vi "Run.vi"(8 "error in (no error)":errorcluster, 11 "Channel GUI in":refnum<class "Channel.lvclass">) -> (0 "error out":errorcluster, 3 "Channel GUI out":refnum<class "Channel.lvclass">)   [LabVIEW 2018, in "Channel.lvclass"]
uses:
  Channel.lvclass
  Channel.lvclass/Channel.ctl
  State Machine/State Machine.lvclass
  Camera/Camera.lvclass
  RxTx/RxTx.lvclass
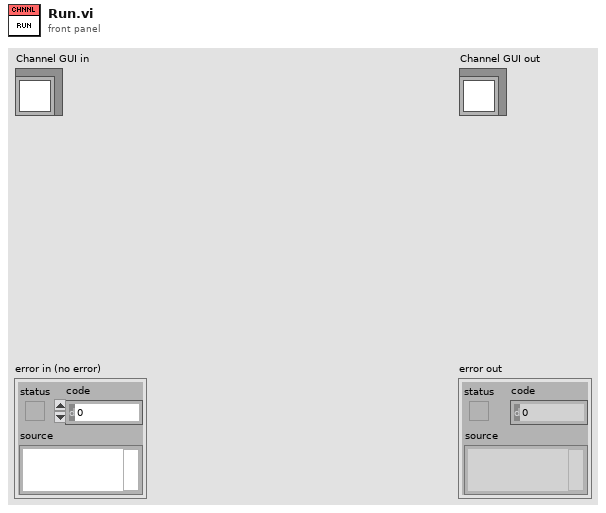
[diagram p1: front panel]
types:
  T1 = cluster{"PREAMP":u16, "READOUT_RATE":u16, "VERTICAL_SHIFT_SPEED":u16, "READ_MODE":u16, "VERTICAL_CLOCK_VOLTAGE":u16, "ACQUISITION_MODE":u16, "AD_CHANNEL":u16, "SHUTTER_TTL":u16, "SHUTTER_OPENING_TIME":u16, "SHUTTER_CLOSING_TIME":u16, "SHUTTER_MODE":u16, "TRIGGER_MODE":u16, "VBIN":u16, "INITIAL_LINE":u16, "INITIAL_COLUMN":u16, "FINAL_LINE":u16, "FINAL_COLUMN":u16, "HBIN":u16}
  T2 = cluster{"EXPTIME":dbl, "#FRAMES":u32, "#CYCLES":u32, "suffix":string, "TEMP":i32, "COOLER_POWER_STATUS":u16}
  T3 = cluster{"CYCLES_DONE":u16, "LAST_IMAGE_NAME":string, "USED_DISK_SPACE":u16, "FRAMES_DONE":u16, "CCD_STATUS":string, "CURRENT_TEMPERATURE":i16, "TEMPERATURE_STATUS":string, "FRAME_EXPOSURE_TIME":sgl, "ERROR":bool, "SERIAL_NUMBER":u16, "ACQUIRING":bool, "IMAGE_INDEX":u32, "power":bool, "acs mode":bool}
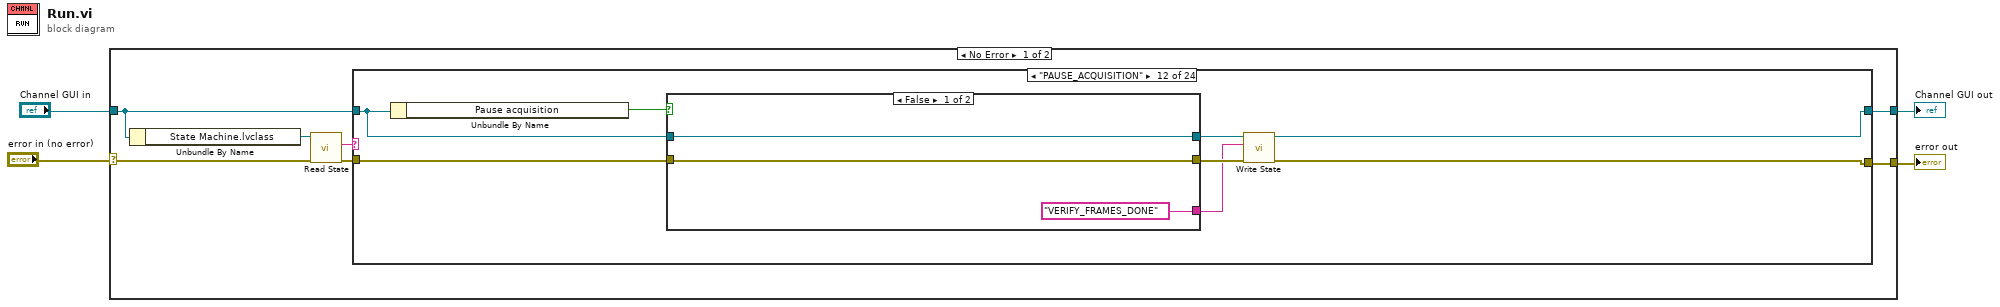
[diagram p0: block diagram]
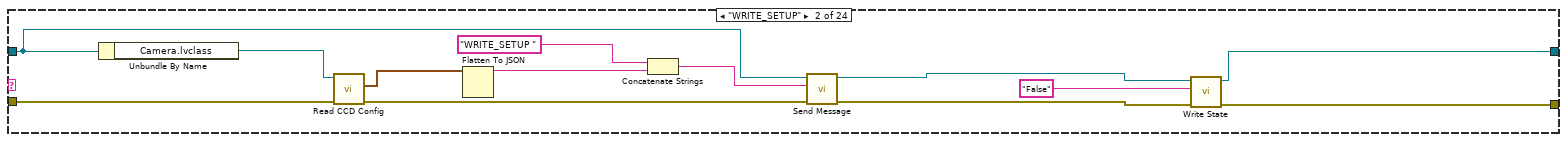
[diagram p3: hidden frame]
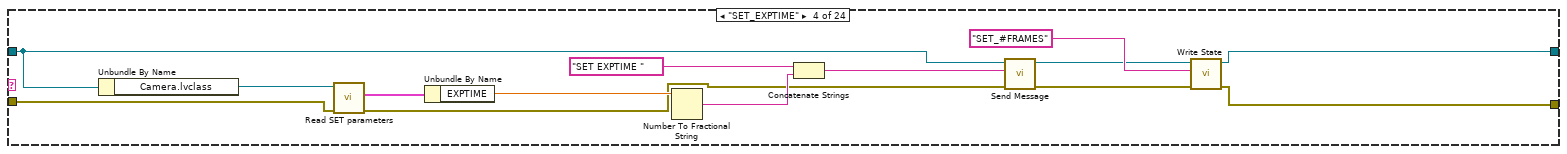
[diagram p5: hidden frame]
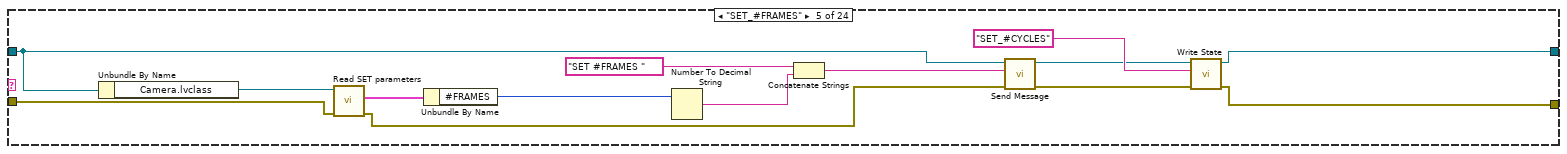
[diagram p6: hidden frame]
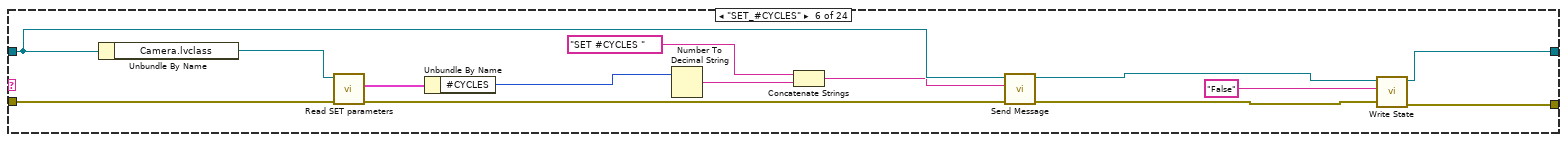
[diagram p7: hidden frame]
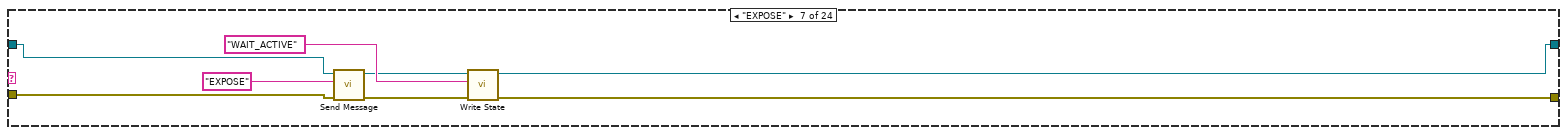
[diagram p8: hidden frame]
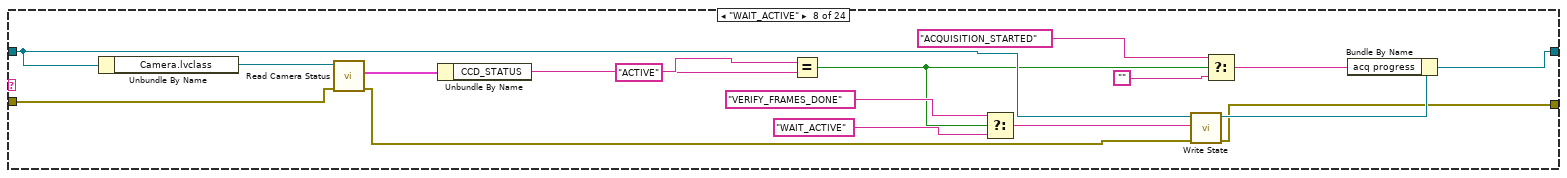
[diagram p9: hidden frame]
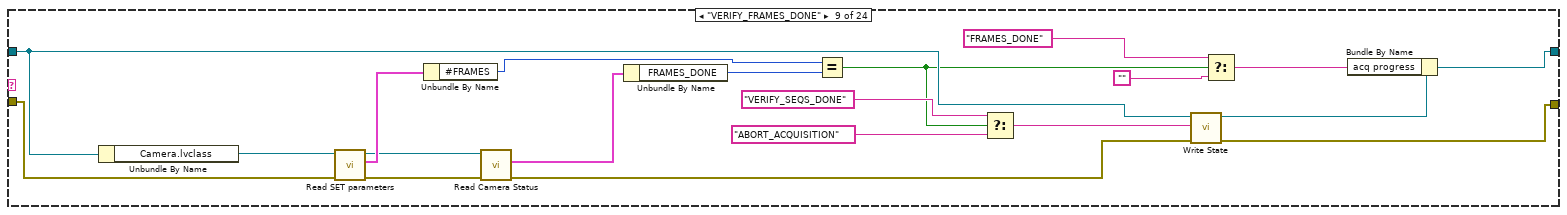
[diagram p10: hidden frame]
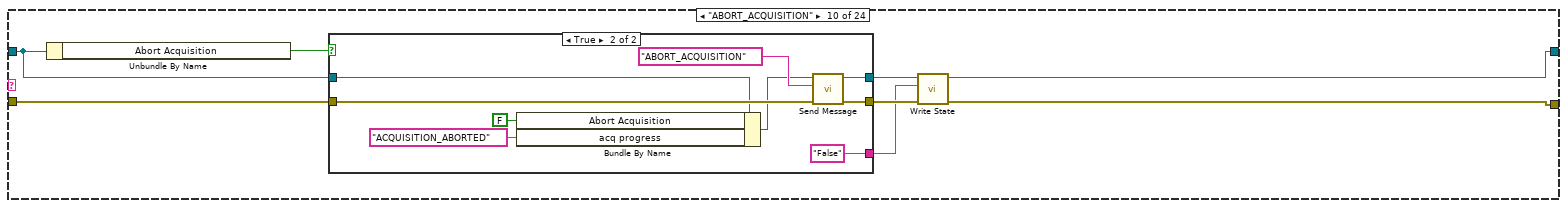
[diagram p11: hidden frame]
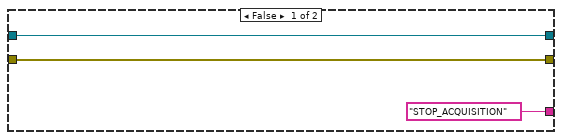
[diagram p12: hidden frame]
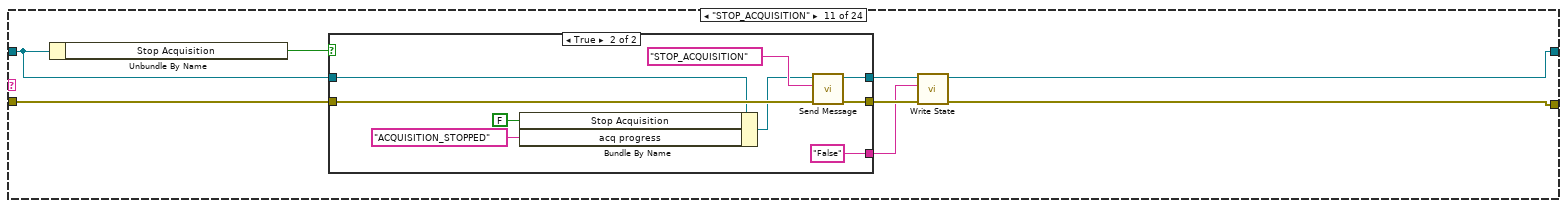
[diagram p13: hidden frame]
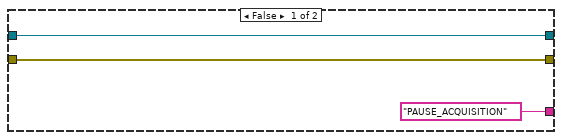
[diagram p14: hidden frame]
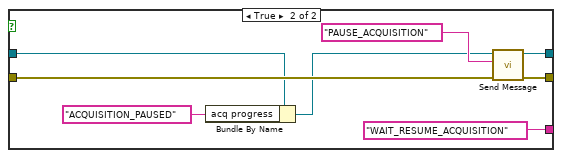
[diagram p15: hidden frame]
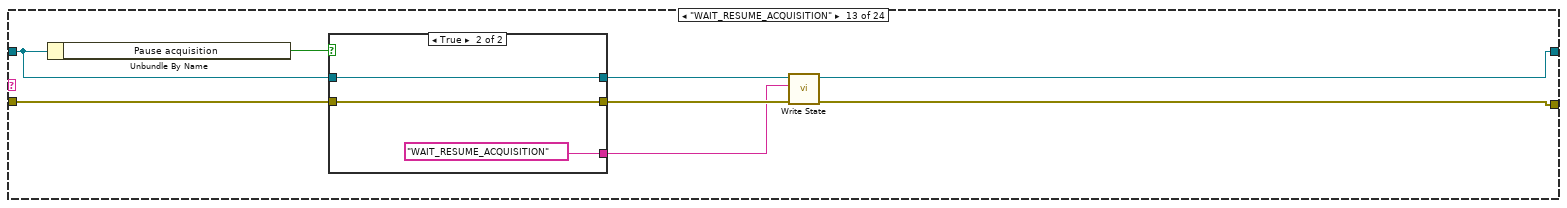
[diagram p16: hidden frame]
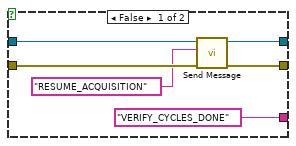
[diagram p17: hidden frame]
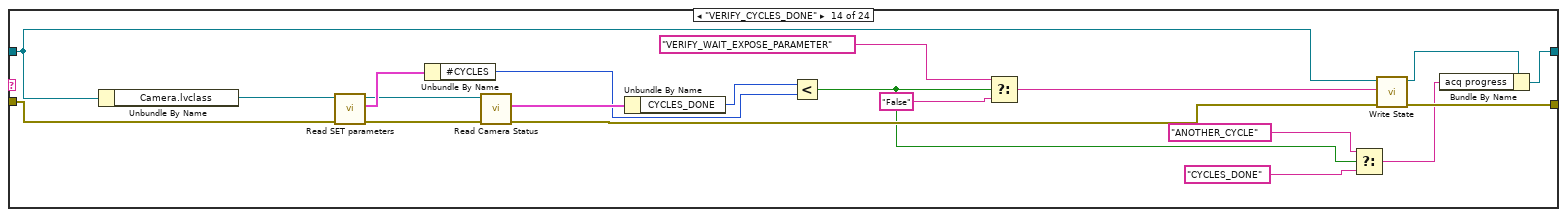
[diagram p18: hidden frame]
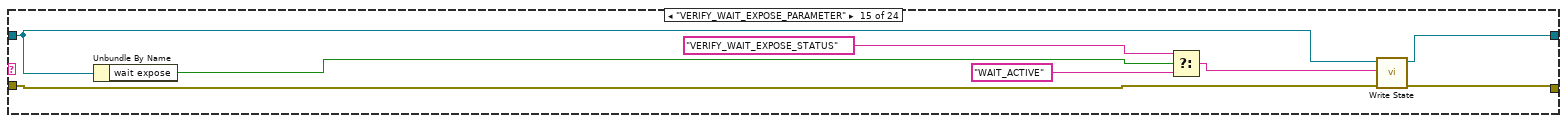
[diagram p19: hidden frame]
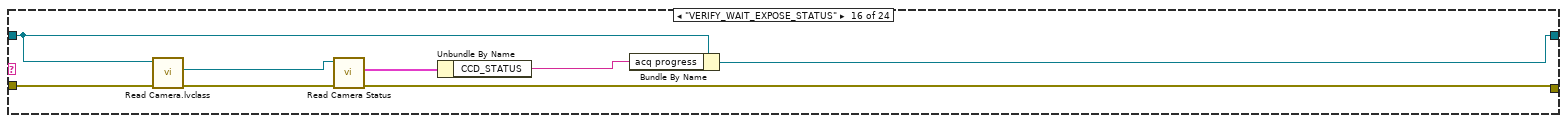
[diagram p20: hidden frame]
diagram:
  n1 = case shown="No Error" "error in (no error)" {
    selector: "error in (no error)" -> [w9 w328]
    tunnel: [w11 w328] -> w2
    tunnel: "Channel GUI in" -> [w7 w327]
    tunnel: [w6 w327] -> w1
    frame No Error {
      n2 = Unbundle By Name(w7) -> ("State Machine.lvclass"=w10:refnum<class "State Machine.lvclass">)
      n3 = call-dynamic "Read State.vi"("error in (no error)"=w9, "State Machine in"=w10) -> ("error out"=w8:errorcluster, "State"=w5:string)  [unwired: 7 in, 1 out]
      n4 = case shown="\"PAUSE_ACQUISITION\"" w5 {
        tunnel: w8 -> [w13 w25 w27 w39 w53 w67 w75 w94 w111 w123 w143 w163 w182 w207 w216 w227 w232 w235 w249 w263 w277 w290 w298 w316]
        tunnel: [w13 w19 w27 w34 w49 w64 w77 w83 w115 w118 w138 w158 w177 w211 w219 w220 w234 w235 w247 w261 w275 w288 w299 w318] -> w11
        tunnel: w7 -> [w12 w16 w28 w31 w47 w59 w76 w86 w102 w121 w141 w161 w180 w201 w215 w223 w230 w236 w245 w259 w273 w284 w295 w314]
        tunnel: [w12 w20 w28 w35 w50 w65 w71 w84 w100 w119 w139 w159 w178 w195 w212 w221 w233 w236 w248 w262 w276 w289 w296 w312] -> w6
        frame "False", Default {
        }
        frame "WRITE_SETUP" {
          n5 = Unbundle By Name(w16) -> ("Camera.lvclass"=w26:refnum<class "Camera.lvclass">)
          n6 = call-dynamic "Read CCD Config.vi"("error in (no error)"=w25, "Camera in"=w26) -> ("error out"=w18:errorcluster, "CCD Config"=w24:T1)  [unwired: 7 in, 1 out]
          n7 = Flatten To JSON(anything=w24) -> (JSON string=w22:string)  [unwired: 2 in, 1 out]
          n8 = Concatenate Strings("WRITE_SETUP ", w22) -> (w14:string)
          n9 = call "Send Message.vi"("error in (no error)"=w18, "Message"=w14, "Channel GUI in"=w16) -> ("error out"=w17:errorcluster, "Channel GUI out"=w15:refnum<class "Channel.lvclass">)  [unwired: 7 in]
          n10 = call "Write State.vi"("error in (no error)"=w17, "State"="False" ("New_State"), "Channel GEI in"=w15) -> ("error out"=w19:errorcluster, "Channel GEI out"=w20:refnum<class "Channel.lvclass">)  [unwired: 7 in]
        }
        frame "--------------------------" {
        }
        frame "SET_EXPTIME" {
          n11 = Unbundle By Name(w31) -> ("Camera.lvclass"=w40:refnum<class "Camera.lvclass">)
          n12 = call-dynamic "Read SET parameters.vi"("error in (no error)"=w39, "Camera in"=w40) -> ("error out"=w33:errorcluster, "SET parameters"=w38:T2)  [unwired: 7 in, 1 out]
          n13 = Unbundle By Name(w38) -> ("EXPTIME"=w37:dbl)
          n14 = Number To Fractional String(number=w37) -> (F-format string=w42:string)  [unwired: 3 in]
          n15 = Concatenate Strings("SET EXPTIME ", w42) -> (w29:string)
          n16 = call "Send Message.vi"("error in (no error)"=w33, "Message"=w29, "Channel GUI in"=w31) -> ("error out"=w32:errorcluster, "Channel GUI out"=w30:refnum<class "Channel.lvclass">)  [unwired: 7 in]
          n17 = call "Write State.vi"("error in (no error)"=w32, "State"="SET_#FRAMES" ("New_State"), "Channel GEI in"=w30) -> ("error out"=w34:errorcluster, "Channel GEI out"=w35:refnum<class "Channel.lvclass">)  [unwired: 7 in]
        }
        frame "SET_#FRAMES" {
          n18 = Unbundle By Name(w47) -> ("Camera.lvclass"=w54:refnum<class "Camera.lvclass">)
          n19 = call-dynamic "Read SET parameters.vi"("error in (no error)"=w53, "Camera in"=w54) -> ("error out"=w44:errorcluster, "SET parameters"=w52:T2)  [unwired: 7 in, 1 out]
          n20 = Unbundle By Name(w52) -> ("#FRAMES"=w51:u32)
          n21 = Number To Decimal String(number=w51) -> (decimal integer string=w56:string)  [unwired: 1 in]
          n22 = Concatenate Strings("SET #FRAMES ", w56) -> (w43:string)
          n23 = call "Send Message.vi"("error in (no error)"=w44, "Message"=w43, "Channel GUI in"=w47) -> ("error out"=w45:errorcluster, "Channel GUI out"=w46:refnum<class "Channel.lvclass">)  [unwired: 7 in]
          n24 = call "Write State.vi"("error in (no error)"=w45, "State"="SET_#CYCLES" ("New_State"), "Channel GEI in"=w46) -> ("error out"=w49:errorcluster, "Channel GEI out"=w50:refnum<class "Channel.lvclass">)  [unwired: 7 in]
        }
        frame "SET_#CYCLES" {
          n25 = Unbundle By Name(w59) -> ("Camera.lvclass"=w68:refnum<class "Camera.lvclass">)
          n26 = call-dynamic "Read SET parameters.vi"("error in (no error)"=w67, "Camera in"=w68) -> ("error out"=w61:errorcluster, "SET parameters"=w66:T2)  [unwired: 7 in, 1 out]
          n27 = Unbundle By Name(w66) -> ("#CYCLES"=w62:u32)
          n28 = Number To Decimal String(number=w62) -> (decimal integer string=w70:string)  [unwired: 1 in]
          n29 = Concatenate Strings("SET #CYCLES ", w70) -> (w57:string)
          n30 = call "Send Message.vi"("error in (no error)"=w61, "Message"=w57, "Channel GUI in"=w59) -> ("error out"=w60:errorcluster, "Channel GUI out"=w58:refnum<class "Channel.lvclass">)  [unwired: 7 in]
          n31 = call "Write State.vi"("error in (no error)"=w60, "State"="False" ("New_State"), "Channel GEI in"=w58) -> ("error out"=w64:errorcluster, "Channel GEI out"=w65:refnum<class "Channel.lvclass">)  [unwired: 7 in]
        }
        frame "EXPOSE" {
          n32 = call "Send Message.vi"("error in (no error)"=w75, "Message"="EXPOSE", "Channel GUI in"=w76) -> ("error out"=w74:errorcluster, "Channel GUI out"=w73:refnum<class "Channel.lvclass">)  [unwired: 7 in]
          n33 = call "Write State.vi"("error in (no error)"=w74, "State"="WAIT_ACTIVE", "Channel GEI in"=w73) -> ("error out"=w77:errorcluster, "Channel GEI out"=w71:refnum<class "Channel.lvclass">)  [unwired: 7 in]
        }
        frame "WAIT_ACTIVE" {
          n34 = Unbundle By Name(w86) -> ("Camera.lvclass"=w95:refnum<class "Camera.lvclass">)
          n35 = call-dynamic "Read Camera Status.vi"("error in (no error)"=w94, "Camera in"=w95) -> ("error out"=w90:errorcluster, "Camera Status"=w93:T3)  [unwired: 7 in, 1 out]
          n36 = Unbundle By Name(w93) -> ("CCD_STATUS"=w92:string)
          n37 = Equal?(x=w92, y="ACTIVE") -> (x = y?=w79:bool)
          n38 = Select(t="VERIFY_FRAMES_DONE" ("y"), s=w79, f="WAIT_ACTIVE" ("y")) -> (s? t:f=w87:string)
          n39 = call "Write State.vi"("error in (no error)"=w90, "State"=w87, "Channel GEI in"=w86) -> ("error out"=w83:errorcluster, "Channel GEI out"=w85:refnum<class "Channel.lvclass">)  [unwired: 7 in]
          n40 = Select(t="ACQUISITION_STARTED" ("y"), s=w79, f="") -> (s? t:f=w82:string)
          n41 = Bundle By Name(cluster=w85, "acq progress"=w82) -> (w84:refnum<class "Channel.lvclass">)
        }
        frame "VERIFY_FRAMES_DONE" {
          n42 = Unbundle By Name(w102) -> ("Camera.lvclass"=w112:refnum<class "Camera.lvclass">)
          n43 = call-dynamic "Read SET parameters.vi"("error in (no error)"=w111, "Camera in"=w112) -> ("error out"=w106:errorcluster, "SET parameters"=w110:T2, "Camera out"=w107:refnum<class "Camera.lvclass">)  [unwired: 7 in]
          n44 = Unbundle By Name(w110) -> ("#FRAMES"=w104:u32)
          n45 = call-dynamic "Read Camera Status.vi"("error in (no error)"=w106, "Camera in"=w107) -> ("error out"=w105:errorcluster, "Camera Status"=w109:T3)  [unwired: 7 in, 1 out]
          n46 = Unbundle By Name(w109) -> ("FRAMES_DONE"=w108:u16)
          n47 = Equal?(x=w104, y=w108) -> (x = y?=w97:bool)
          n48 = Select(t="VERIFY_SEQS_DONE" ("Message"), s=w97, f="ABORT_ACQUISITION" ("Message")) -> (s? t:f=w113:string)
          n49 = call "Write State.vi"("error in (no error)"=w105, "State"=w113, "Channel GEI in"=w102) -> ("error out"=w115:errorcluster, "Channel GEI out"=w101:refnum<class "Channel.lvclass">)  [unwired: 7 in]
          n50 = Select(t="FRAMES_DONE" ("Message"), s=w97, f="") -> (s? t:f=w99:string)
          n51 = Bundle By Name(cluster=w101, "acq progress"=w99) -> (w100:refnum<class "Channel.lvclass">)
        }
        frame "ABORT_ACQUISITION" {
          n52 = Unbundle By Name(w121) -> ("Abort Acquisition"=w122:bool)
          n53 = case shown="True" w122 {
            tunnel: [w125 w132] -> w117
            tunnel: [w126 w133] -> w120
            tunnel: w121 -> [w126 w130]
            tunnel: w123 -> [w125 w135]
            tunnel: ["STOP_ACQUISITION" ("Message") "False" ("Message")] -> w116
            frame False {
            }
            frame True {
              n54 = Bundle By Name(cluster=w130, "Abort Acquisition"=FALSE ("prev acquisition control.Abort Acquisition"), "acq progress"="ACQUISITION_ABORTED") -> (w129:refnum<class "Channel.lvclass">)
              n55 = call "Send Message.vi"("error in (no error)"=w135, "Message"="ABORT_ACQUISITION", "Channel GUI in"=w129) -> ("error out"=w132:errorcluster, "Channel GUI out"=w133:refnum<class "Channel.lvclass">)  [unwired: 7 in]
            }
          }
          n56 = call "Write State.vi"("error in (no error)"=w117, "State"=w116, "Channel GEI in"=w120) -> ("error out"=w118:errorcluster, "Channel GEI out"=w119:refnum<class "Channel.lvclass">)  [unwired: 7 in]
        }
        frame "STOP_ACQUISITION" {
          n57 = Unbundle By Name(w141) -> ("Stop Acquisition"=w142:bool)
          n58 = case shown="True" w142 {
            tunnel: [w145 w152] -> w137
            tunnel: [w146 w153] -> w140
            tunnel: w141 -> [w146 w150]
            tunnel: w143 -> [w145 w155]
            tunnel: ["PAUSE_ACQUISITION" ("Message") "False" ("Message")] -> w136
            frame False {
            }
            frame True {
              n59 = Bundle By Name(cluster=w150, "Stop Acquisition"=FALSE ("prev acquisition control.Abort Acquisition"), "acq progress"="ACQUISITION_STOPPED") -> (w149:refnum<class "Channel.lvclass">)
              n60 = call "Send Message.vi"("error in (no error)"=w155, "Message"="STOP_ACQUISITION", "Channel GUI in"=w149) -> ("error out"=w152:errorcluster, "Channel GUI out"=w153:refnum<class "Channel.lvclass">)  [unwired: 7 in]
            }
          }
          n61 = call "Write State.vi"("error in (no error)"=w137, "State"=w136, "Channel GEI in"=w140) -> ("error out"=w138:errorcluster, "Channel GEI out"=w139:refnum<class "Channel.lvclass">)  [unwired: 7 in]
        }
        frame "PAUSE_ACQUISITION" {
          n62 = Unbundle By Name(w161) -> ("Pause acquisition"=w162:bool)
          n63 = case shown="False" w162 {
            tunnel: [w165 w171] -> w157
            tunnel: [w166 w172] -> w160
            tunnel: w161 -> [w166 w169]
            tunnel: w163 -> [w165 w174]
            tunnel: ["VERIFY_FRAMES_DONE" ("Message") "WAIT_RESUME_ACQUISITION" ("Message")] -> w156
            frame False {
            }
            frame True {
              n64 = Bundle By Name(cluster=w169, "acq progress"="ACQUISITION_PAUSED") -> (w168:refnum<class "Channel.lvclass">)
              n65 = call "Send Message.vi"("error in (no error)"=w174, "Message"="PAUSE_ACQUISITION", "Channel GUI in"=w168) -> ("error out"=w171:errorcluster, "Channel GUI out"=w172:refnum<class "Channel.lvclass">)  [unwired: 7 in]
            }
          }
          n66 = call "Write State.vi"("error in (no error)"=w157, "State"=w156, "Channel GEI in"=w160) -> ("error out"=w158:errorcluster, "Channel GEI out"=w159:refnum<class "Channel.lvclass">)  [unwired: 7 in]
        }
        frame "WAIT_RESUME_ACQUISITION" {
          n67 = Unbundle By Name(w180) -> ("Pause acquisition"=w181:bool)
          n68 = case shown="True" w181 {
            tunnel: [w185 w190] -> w176
            tunnel: [w186 w191] -> w179
            tunnel: w180 -> [w184 w191]
            tunnel: w182 -> [w188 w190]
            tunnel: ["VERIFY_CYCLES_DONE" ("Message") "WAIT_RESUME_ACQUISITION" ("Message")] -> w175
            frame False {
              n69 = call "Send Message.vi"("error in (no error)"=w188, "Message"="RESUME_ACQUISITION", "Channel GUI in"=w184) -> ("error out"=w185:errorcluster, "Channel GUI out"=w186:refnum<class "Channel.lvclass">)  [unwired: 7 in]
            }
            frame True {
            }
          }
          n70 = call "Write State.vi"("error in (no error)"=w176, "State"=w175, "Channel GEI in"=w179) -> ("error out"=w177:errorcluster, "Channel GEI out"=w178:refnum<class "Channel.lvclass">)  [unwired: 7 in]
        }
        frame "VERIFY_CYCLES_DONE" {
          n71 = Unbundle By Name(w201) -> ("Camera.lvclass"=w208:refnum<class "Camera.lvclass">)
          n72 = call-dynamic "Read SET parameters.vi"("error in (no error)"=w207, "Camera in"=w208) -> ("error out"=w203:errorcluster, "SET parameters"=w206:T2, "Camera out"=w204:refnum<class "Camera.lvclass">)  [unwired: 7 in]
          n73 = Unbundle By Name(w206) -> ("#CYCLES"=w198:u32)
          n74 = call-dynamic "Read Camera Status.vi"("error in (no error)"=w203, "Camera in"=w204) -> ("error out"=w202:errorcluster, "Camera Status"=w205:T3)  [unwired: 7 in, 1 out]
          n75 = Unbundle By Name(w205) -> ("CYCLES_DONE"=w199:u16)
          n76 = Less?(x=w199, y=w198) -> (x < y?=w192:bool)
          n77 = Select(t="VERIFY_WAIT_EXPOSE_PARAMETER" ("Message"), s=w192, f="False" ("Message")) -> (s? t:f=w209:string)
          n78 = Select(t="ANOTHER_CYCLE" ("y"), s=w192, f="CYCLES_DONE" ("y")) -> (s? t:f=w194:string)
          n79 = call "Write State.vi"("error in (no error)"=w202, "State"=w209, "Channel GEI in"=w201) -> ("error out"=w211:errorcluster, "Channel GEI out"=w196:refnum<class "Channel.lvclass">)  [unwired: 7 in]
          n80 = Bundle By Name(cluster=w196, "acq progress"=w194) -> (w195:refnum<class "Channel.lvclass">)
        }
        frame "VERIFY_WAIT_EXPOSE_PARAMETER" {
          n81 = Unbundle By Name(w215) -> ("wait expose"=w213:bool)
          n82 = Select(t="VERIFY_WAIT_EXPOSE_STATUS" ("Message"), s=w213, f="WAIT_ACTIVE" ("Message")) -> (s? t:f=w217:string)
          n83 = call "Write State.vi"("error in (no error)"=w216, "State"=w217, "Channel GEI in"=w215) -> ("error out"=w219:errorcluster, "Channel GEI out"=w212:refnum<class "Channel.lvclass">)  [unwired: 7 in]
        }
        frame "VERIFY_WAIT_EXPOSE_STATUS" {
          n84 = call-dynamic "Read Camera.lvclass.vi"("error in (no error)"=w227, "Channel in"=w223) -> ("error out"=w225:errorcluster, "Camera.lvclass"=w226:refnum<class "Camera.lvclass">)  [unwired: 7 in, 1 out]
          n85 = call-dynamic "Read Camera Status.vi"("error in (no error)"=w225, "Camera in"=w226) -> ("error out"=w220:errorcluster, "Camera Status"=w224:T3)  [unwired: 7 in, 1 out]
          n86 = Unbundle By Name(w224) -> ("CCD_STATUS"=w222:string)
          n87 = Bundle By Name(cluster=w223, "acq progress"=w222) -> (w221:refnum<class "Channel.lvclass">)
        }
        frame "WRITE_ACQUISITION_FINISHED" {
          n88 = Bundle By Name(cluster=w230, "acq finished"=TRUE) -> (w231:refnum<class "Channel.lvclass">)
          n89 = call "Write State.vi"("error in (no error)"=w232, "State"="False", "Channel GEI in"=w231) -> ("error out"=w234:errorcluster, "Channel GEI out"=w233:refnum<class "Channel.lvclass">)  [unwired: 7 in]
        }
        frame "-----------------------------------" {
        }
        frame "SET_SUFFIX" {
          n90 = Unbundle By Name(w245) -> ("Camera.lvclass"=w240:refnum<class "Camera.lvclass">)
          n91 = call-dynamic "Read SET parameters.vi"("error in (no error)"=w249, "Camera in"=w240) -> ("error out"=w242:errorcluster, "SET parameters"=w239:T2)  [unwired: 7 in, 1 out]
          n92 = Unbundle By Name(w239) -> ("suffix"=w237:string)
          n93 = Concatenate Strings("SET SUFFIX ", w237) -> (w241:string)
          n94 = call "Send Message.vi"("error in (no error)"=w242, "Message"=w241, "Channel GUI in"=w245) -> ("error out"=w243:errorcluster, "Channel GUI out"=w244:refnum<class "Channel.lvclass">)  [unwired: 7 in]
          n95 = call "Write State.vi"("error in (no error)"=w243, "State"="False", "Channel GEI in"=w244) -> ("error out"=w247:errorcluster, "Channel GEI out"=w248:refnum<class "Channel.lvclass">)  [unwired: 7 in]
        }
        frame "SET_COOLER" {
          n96 = Unbundle By Name(w259) -> ("Camera.lvclass"=w254:refnum<class "Camera.lvclass">)
          n97 = call-dynamic "Read SET parameters.vi"("error in (no error)"=w263, "Camera in"=w254) -> ("error out"=w256:errorcluster, "SET parameters"=w253:T2)  [unwired: 7 in, 1 out]
          n98 = Unbundle By Name(w253) -> ("COOLER_POWER_STATUS"=w251:u16)
          n99 = Number To Decimal String(number=w251) -> (decimal integer string=w250:string)  [unwired: 1 in]
          n100 = Concatenate Strings("SET COOLER_POWER_STATUS ", w250) -> (w255:string)
          n101 = call "Send Message.vi"("error in (no error)"=w256, "Message"=w255, "Channel GUI in"=w259) -> ("error out"=w257:errorcluster, "Channel GUI out"=w258:refnum<class "Channel.lvclass">)  [unwired: 7 in]
          n102 = call "Write State.vi"("error in (no error)"=w257, "State"="False", "Channel GEI in"=w258) -> ("error out"=w261:errorcluster, "Channel GEI out"=w262:refnum<class "Channel.lvclass">)  [unwired: 7 in]
        }
        frame "SET_TEMP" {
          n103 = Unbundle By Name(w273) -> ("Camera.lvclass"=w268:refnum<class "Camera.lvclass">)
          n104 = call-dynamic "Read SET parameters.vi"("error in (no error)"=w277, "Camera in"=w268) -> ("error out"=w270:errorcluster, "SET parameters"=w267:T2)  [unwired: 7 in, 1 out]
          n105 = Unbundle By Name(w267) -> ("TEMP"=w265:i32)
          n106 = Number To Decimal String(number=w265) -> (decimal integer string=w264:string)  [unwired: 1 in]
          n107 = Concatenate Strings("SET TEMP ", w264) -> (w269:string)
          n108 = call "Send Message.vi"("error in (no error)"=w270, "Message"=w269, "Channel GUI in"=w273) -> ("error out"=w271:errorcluster, "Channel GUI out"=w272:refnum<class "Channel.lvclass">)  [unwired: 7 in]
          n109 = call "Write State.vi"("error in (no error)"=w271, "State"="False", "Channel GEI in"=w272) -> ("error out"=w275:errorcluster, "Channel GEI out"=w276:refnum<class "Channel.lvclass">)  [unwired: 7 in]
        }
        frame "SET_WAIT_EXPOSE_COMMAND" {
          n110 = Unbundle By Name(w284) -> ("wait expose"=w278:bool)
          n111 = Select(t="ON", s=w278, f="OFF") -> (s? t:f=w280:string)
          n112 = Concatenate Strings("WAIT_EXPOSE_COMMAND ", w280) -> (w281:string)
          n113 = call "Send Message.vi"("error in (no error)"=w290, "Message"=w281, "Channel GUI in"=w284) -> ("error out"=w285:errorcluster, "Channel GUI out"=w286:refnum<class "Channel.lvclass">)  [unwired: 7 in]
          n114 = call "Write State.vi"("error in (no error)"=w285, "State"="False", "Channel GEI in"=w286) -> ("error out"=w288:errorcluster, "Channel GEI out"=w289:refnum<class "Channel.lvclass">)  [unwired: 7 in]
        }
        frame "WAIT" {
          n115 = Unbundle By Name(w295) -> ("State Machine.lvclass"=w293:refnum<class "State Machine.lvclass">)
          n116 = call "Verify Timer.vi"("error in (no error)"=w298, "State Machine in"=w293) -> ("error out"=w297:errorcluster, "time out"=w291:bool, "State Machine out"=w292:refnum<class "State Machine.lvclass">)  [unwired: 7 in]
          n117 = Bundle By Name(cluster=w295, "State Machine.lvclass"=w292) -> (w294:refnum<class "Channel.lvclass">)
          n118 = case shown="True" w291 {
            tunnel: [w300 w307] -> w299
            tunnel: w297 -> [w300 w305]
            tunnel: [w301 w303] -> w296
            tunnel: w294 -> [w301 w302]
            frame False {
            }
            frame True {
              n119 = Unbundle By Name(w302) -> ("State Machine.lvclass"=w304:refnum<class "State Machine.lvclass">)
              n120 = call "Set Next State.vi"("error in (no error)"=w305, "State Machine in"=w304) -> ("error out"=w307:errorcluster, "State Machine out"=w306:refnum<class "State Machine.lvclass">)  [unwired: 8 in]
              n121 = Bundle By Name(cluster=w302, "State Machine.lvclass"=w306) -> (w303:refnum<class "Channel.lvclass">)
            }
          }
        }
        frame "WAIT_DONE" {
          n122 = Unbundle By Name(w314) -> ("RxTx.lvclass"=w317:refnum<class "RxTx.lvclass">)
          n123 = call "Read Rx Command.vi"("error in (no error)"=w316, "RxTx in"=w317) -> ("error out"=w310:errorcluster, "Rx Command"=w315:string, "RxTx out"=w311:refnum<class "RxTx.lvclass">)  [unwired: 7 in]
          n124 = Bundle By Name(cluster=w314, "RxTx.lvclass"=w311) -> (w313:refnum<class "Channel.lvclass">)
          n125 = Equal?(x=w315, y="DONE") -> (x = y?=w308:bool)
          n126 = case shown="True" w308 {
            tunnel: [w319 w326] -> w318
            tunnel: w313 -> [w320 w323]
            tunnel: [w320 w322] -> w312
            tunnel: w310 -> [w319 w321]
            frame False {
            }
            frame True {
              n127 = Unbundle By Name(w323) -> ("State Machine.lvclass"=w324:refnum<class "State Machine.lvclass">)
              n128 = call "Set Next State.vi"("error in (no error)"=w321, "State Machine in"=w324) -> ("error out"=w326:errorcluster, "State Machine out"=w325:refnum<class "State Machine.lvclass">)  [unwired: 8 in]
              n129 = Bundle By Name(cluster=w323, "State Machine.lvclass"=w325) -> (w322:refnum<class "Channel.lvclass">)
            }
          }
        }
      }
    }
    frame Error {
    }
  }
  "error out" <- w2
  "Channel GUI out" <- w1
